vi "Get visa 1d DBL data.vi"(7 "VISA resource name":refnum<visa-resource-name>, 8 "error in (no error)":errorcluster, 9 "Name":string, 10 "Mag Lab Parameters in":refnum<class "Mag Lab Parameters.lvclass">, 11 "Stanford Research in":refnum<class "Stanford Research.lvclass">) -> (0 "error out":errorcluster, 1 "Channel data":dbl[](array[numeric]), 2 "Channel names":string[](array[string]), 3 "Stanford Research out":refnum<class "Stanford Research.lvclass">, 5 "VISA resource name out":refnum<visa-resource-name>)   [LabVIEW 2015, in "Stanford Research.lvclass"]
uses:
  Stanford Research.lvclass
  Mag Lab Properties/Mag Lab Parameters.lvclass
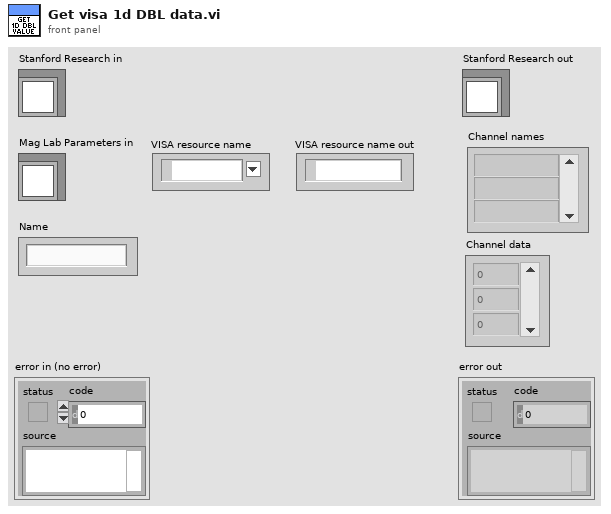
[diagram p1: front panel]
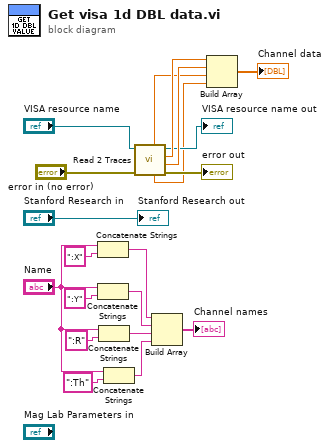
[diagram p0: block diagram]
diagram:
  n1 = Concatenate Strings("Name", ":X" ("string")) -> (w11:string)
  n2 = Concatenate Strings("Name", ":Y" ("string")) -> (w10:string)
  n3 = Concatenate Strings("Name", ":R" ("string")) -> (w4:string)
  n4 = Concatenate Strings("Name", ":Th" ("string")) -> (w3:string)
  n5 = call "Read 2 Traces.vi"("error in (no error)"="error in (no error)", "VISA Resource Name"="VISA resource name") -> ("error out"=→"error out":errorcluster, "Y"=w17:dbl, "X"=w18:dbl, "VISA Resource Name Out"=→"VISA resource name out":refnum<visa-resource-name>, "theta"=w1:dbl, "r"=w2:dbl)  [unwired: 4 out]
  n6 = Build Array(w11, w10, w4, w3) -> (→"Channel names":string[])
  n7 = Build Array(w18, w17, w2, w1) -> (→"Channel data":dbl[])
  "Stanford Research out" <- "Stanford Research in"
